vi "속도에 따른 라이다 인식 각도범위 찾기.vi"(3 "speed(platform)":dbl) -> (0 "Safe Distance":dbl, 1 "Interested angle":dbl)   [LabVIEW 2016]
uses:
  <vilib>/imath/engines/lvmath2/RunTimeEngine/NodeEndStatement/NIMS_NodeEndStatement_Output.vi
  <instcachedir>/0/NIMS_NodeEndStatement_Output_53EC0D466D134D7ABD903AC30B43404B.lvgen/NIMS_NodeEndStatement_Output_53EC0D466D134D7ABD903AC30B43404B_001.vi
  <instcachedir>/0/NIMS_NodeEndStatement_Output_53EC0D466D134D7ABD903AC30B43404B.lvgen/NIMS_NodeEndStatement_Output_53EC0D466D134D7ABD903AC30B43404B_009.vi
  <vilib>/imath/engines/lvmath2/RunTimeEngine/ErrorHandling/NIMS_Finalize Error.vi
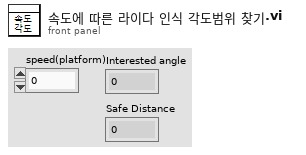
[diagram p1: front panel]
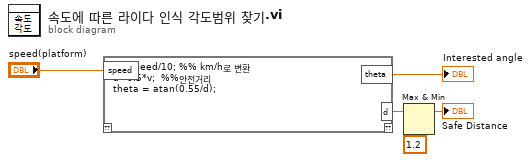
[diagram p0: block diagram]
diagram:
  n1 = mathscript code="v= speed/10; %% km/h로 변환\nd=0.5*v;  %%안전거리\ntheta = atan(0.55/d);"("speed"="speed(platform)") -> ("theta"=→"Interested angle":cdb, "d"=w1:dbl)  [unwired: 1 in, 1 out]
  n2 = Max & Min(x=w1, y=1.2) -> (max(x,y)=→"Safe Distance":dbl)  [unwired: 1 out]
